vi "current_point_info.vi"(0 "pieceOfWorld":T6[][](array[typedef])) -> (1 "foodAmount":T5, 2 "anthillType":T4, 3 "marksArray":T1[](array[typedef]))   [LabVIEW 2015, in "Igor.lvclass"]
uses:
  Igor.lvclass
  actors/world/typedefs/worldCell_cluster.ctl
  actors/world/typedefs/markValue_cluster.ctl
  actors/world/typedefs/markValue.ctl
  actors/world/typedefs/markVolume.ctl
  actors/world/typedefs/amountOfFood.ctl
  actors/world/typedefs/anthillType_enum.ctl
  actors/world/world.lvlib
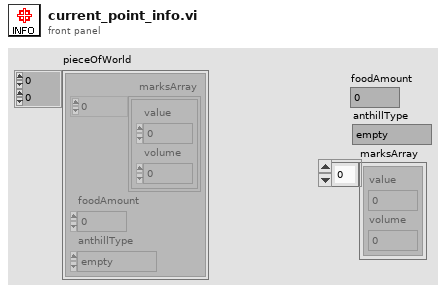
[diagram p1: front panel]
types:
  T1 = typedef "world.lvlib/markValue_cluster.ctl" = cluster{"value":T2, "volume":T3}
  T2 = typedef "world.lvlib/markValue.ctl" = u8
  T3 = typedef "world.lvlib/markVolume.ctl" = u16
  T4 = typedef "world.lvlib/anthillType_enum.ctl" = enum16{"empty", "own", "rival"}
  T5 = typedef "world.lvlib/amountOfFood.ctl" = i32
  T6 = typedef "world.lvlib/worldCell_cluster.ctl" = cluster{"marksArray":T1[], "foodAmount":T5, "anthillType":T4}
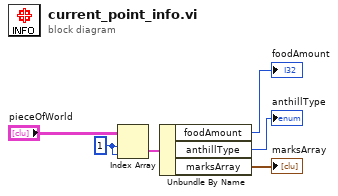
[diagram p0: block diagram]
diagram:
  w6 = 1 ("index (row)")
  n1 = Index Array(array="pieceOfWorld", index (row)=w6, index (col)=w6) -> (element=w5:T6)
  n2 = Unbundle By Name(w5) -> ("foodAmount"=→"foodAmount":T5, "anthillType"=→"anthillType":T4, "marksArray"=→"marksArray":T1[])
